vi "changeRedRatio.vi"(8 "error in (no error)":errorcluster, 9 "Settings":T1={"max velocity"={"Value"=0.0, "Min"=0.0, "Max"=0.0, "StepSize"=0.0, "Tolerance"=0.0, "valueactual"=0.0}, "continious velocity"={"Value"=0.0, "Min"=0.0, "Max"=0.0, "StepSize"=0.0, "Tolerance"=0.0, "valueactual"=0.0}, "shake"=enum."off", "direction"=enum."left", "RedRatio"={"Value"=0.0, "Min"=0.0, "Max"=0.0, "StepSize"=0.0, "Tolerance"=0.0, "valueactual"=0.0}, "StepSize"={"Value"=0.0, "Min"=0.0, "Max"=0.0, "StepSize"=0.0, "Tolerance"=0.0, "valueactual"=0.0}, "position"={"Value"=0.0, "Min"=0.0, "Max"=0.0, "StepSize"=0.0, "Tolerance"=0.0, "valueactual"=0.0}, "velocity"={"Value"=0.0, "Min"=0.0, "Max"=0.0, "StepSize"=0.0, "Tolerance"=0.0, "valueactual"=0.0}, "Step"=enum."off", "Mode"=enum."on demand", "timeout"={"Value"=0.0, "Min"=0.0, "Max"=0.0, "StepSize"=0.0, "Tolerance"=0.0, "valueactual"=0.0}, "DelayStage"={"Value"=0.0, "Min"=0.0, "Max"=0.0, "StepSize"=0.0, "Tolerance"=0.0, "valueactual"=0.0}, "TapeMotor"=enum."off", "encoder Axis"=2, "oldpos"=0.0, "ResetEncoder"=enum."off"}, 10 "NewVal":dbl, 11 "VISA Refnum in":refnum<visa-resource-name>) -> (0 "error out":errorcluster, 1 "Settings":T1={"max velocity"={"Value"=0.0, "Min"=0.0, "Max"=0.0, "StepSize"=0.0, "Tolerance"=0.0, "valueactual"=0.0}, "continious velocity"={"Value"=0.0, "Min"=0.0, "Max"=0.0, "StepSize"=0.0, "Tolerance"=0.0, "valueactual"=0.0}, "shake"=enum."off", "direction"=enum."left", "RedRatio"={"Value"=0.0, "Min"=0.0, "Max"=0.0, "StepSize"=0.0, "Tolerance"=0.0, "valueactual"=0.0}, "StepSize"={"Value"=0.0, "Min"=0.0, "Max"=0.0, "StepSize"=0.0, "Tolerance"=0.0, "valueactual"=0.0}, "position"={"Value"=0.0, "Min"=0.0, "Max"=0.0, "StepSize"=0.0, "Tolerance"=0.0, "valueactual"=0.0}, "velocity"={"Value"=0.0, "Min"=0.0, "Max"=0.0, "StepSize"=0.0, "Tolerance"=0.0, "valueactual"=0.0}, "Step"=enum."off", "Mode"=enum."on demand", "timeout"={"Value"=0.0, "Min"=0.0, "Max"=0.0, "StepSize"=0.0, "Tolerance"=0.0, "valueactual"=0.0}, "DelayStage"={"Value"=0.0, "Min"=0.0, "Max"=0.0, "StepSize"=0.0, "Tolerance"=0.0, "valueactual"=0.0}, "TapeMotor"=enum."off", "encoder Axis"=2, "oldpos"=0.0, "ResetEncoder"=enum."off"}, 2 "redRatio out":dbl, 3 "VISA Refnum out":refnum<visa-resource-name>, 4 "Position (units)":dbl)   [LabVIEW 2011]
uses:
  TapeDrive/settings_TypDef.ctl
  shared/numericVariable_TypeDef.ctl
  shared/OnOffTypeDef.ctl
  TapeDrive/Direction_TypDef.ctl
  TapeDrive/Mode_TypDEf.ctl
  <instrlib>/Newport ESP301/Newport ESP301.lvlib
  TapeDrive/TapeDrive.lvclass
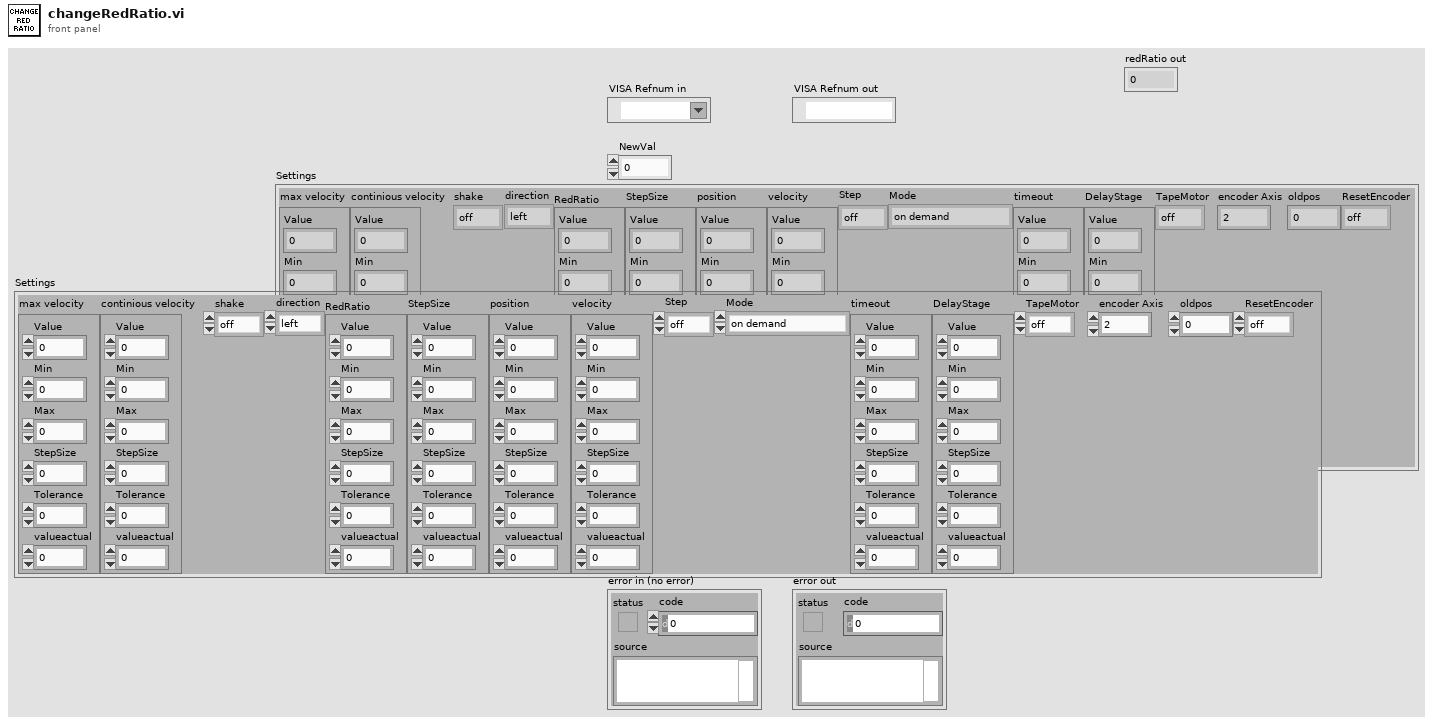
[diagram p1: front panel]
types:
  T1 = typedef "TapeDrive.lvclass/settings_TypDef.ctl" = cluster{"max velocity":T2, "continious velocity":T2, "shake":T3, "direction":T4, "RedRatio":T2, "StepSize":T2, "position":T2, "velocity":T2, "Step":T3, "Mode":T5, "timeout":T2, "DelayStage":T2, "TapeMotor":T3, "encoder Axis":i32, "oldpos":dbl, "ResetEncoder":T3}
  T2 = typedef "numericVariable_TypeDef.ctl" = cluster{"Value":dbl, "Min":dbl, "Max":dbl, "StepSize":dbl, "Tolerance":dbl, "valueactual":dbl}
  T3 = typedef "OnOffTypeDef.ctl" = enum16{"off", "on"}
  T4 = typedef "Direction_TypDef.ctl" = enum16{"left", "right"}
  T5 = typedef "Mode_TypDEf.ctl" = enum16{"on demand", "continuous", "scan"}
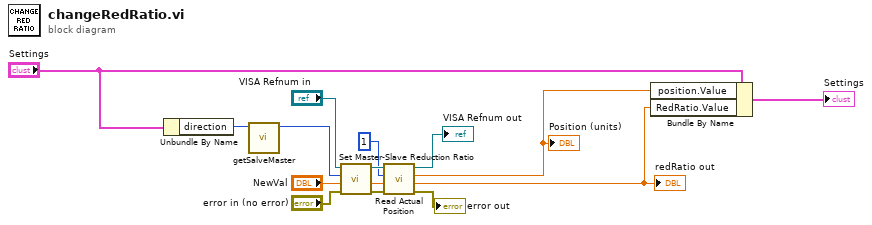
[diagram p0: block diagram]
diagram:
  n1 = Unbundle By Name("Settings") -> ("direction"=w9:T4)
  n2 = call "getSalveMaster.vi"("direction"=w9) -> ("Slave"=w10:i32)  [unwired: 9 in, 1 out]
  n3 = call <instrlib>:"Set Master-Slave Reduction Ratio.vi"("error in (no error)"="error in (no error)", "Reduction Ratio (0)"="NewVal", "Axis (1)"=w10, "VISA resource name"="VISA Refnum in") -> ("error out"=w7:errorcluster, "VISA resource name out"=w5:refnum<visa-resource-name>)  [unwired: 2 in]
  n4 = call <instrlib>:"Read Actual Position.vi"("error in (no error)"=w7, "Axis (1)"=1, "VISA resource name"=w5) -> ("error out"=→"error out":errorcluster, "Position (units)"=w12:dbl, "VISA resource name out"=→"VISA Refnum out":refnum<visa-resource-name>)  [unwired: 2 in]
  "Position (units)" <- w12
  n5 = Bundle By Name(cluster="Settings", "position.Value"=w12, "RedRatio.Value"="NewVal") -> (→"Settings":T1)
  "redRatio out" <- "NewVal"
